vi "Andor_load_xml.vi"(8 "error in":errorcluster, 10 "child node in":refnum<k20>) -> (0 "error out":errorcluster, 2 "child node out":refnum<k20>, 3 "Andor settings":T1)   [LabVIEW 2012]
doc: "Loads HSDIO settings from xml. Expected format:\n\n<EnableHSDIOPulses>%b</EnableHSDIOPulses>\n<ResourceName>%s</ResourceName>\n<ClockRate>%f</ClockRate>\n<unitsPerSecond>%f</unitsPerSecond>\n<HardwareAlignmentQuantum units=\"samples\">%u</HardwareAlignmentQuantum>\n<ArrayOfScriptTriggers columns=\"id, source, type, edge, level\">\n<trigger>%s\\t%s\\t%s\\t%s\\t%s</trigger>\n</ArrayOfScriptTriggers>\n<ChannelsControl columns=\"Description, Active?, Idle State\">\n<channel>%s</channel>\n</ChannelsControl>\n<PulseGenerationScript>%s</PulseGenerationScript>\n<DirectoryToLookForWaveformFiles>%s</DirectoryToLookForWaveformFiles>\n<StartTrigger.WaitForStartTrigger>%b</StartTrigger.WaitForStartTrigger>\n<StartTrigger.source>%s</StartTrigger.source>\n<StartTrigger.edge>%s</StartTrigger.edge>\n\nMTL 2013 Jan 1"
uses:
  Camera/Andor/Andor_settings.ctl
  <vilib>/xml/Close Reference(Node).vi
  <resource>/objmgr/DOMUserDefRef.rc
  <vilib>/xml/NI_XML.lvlib
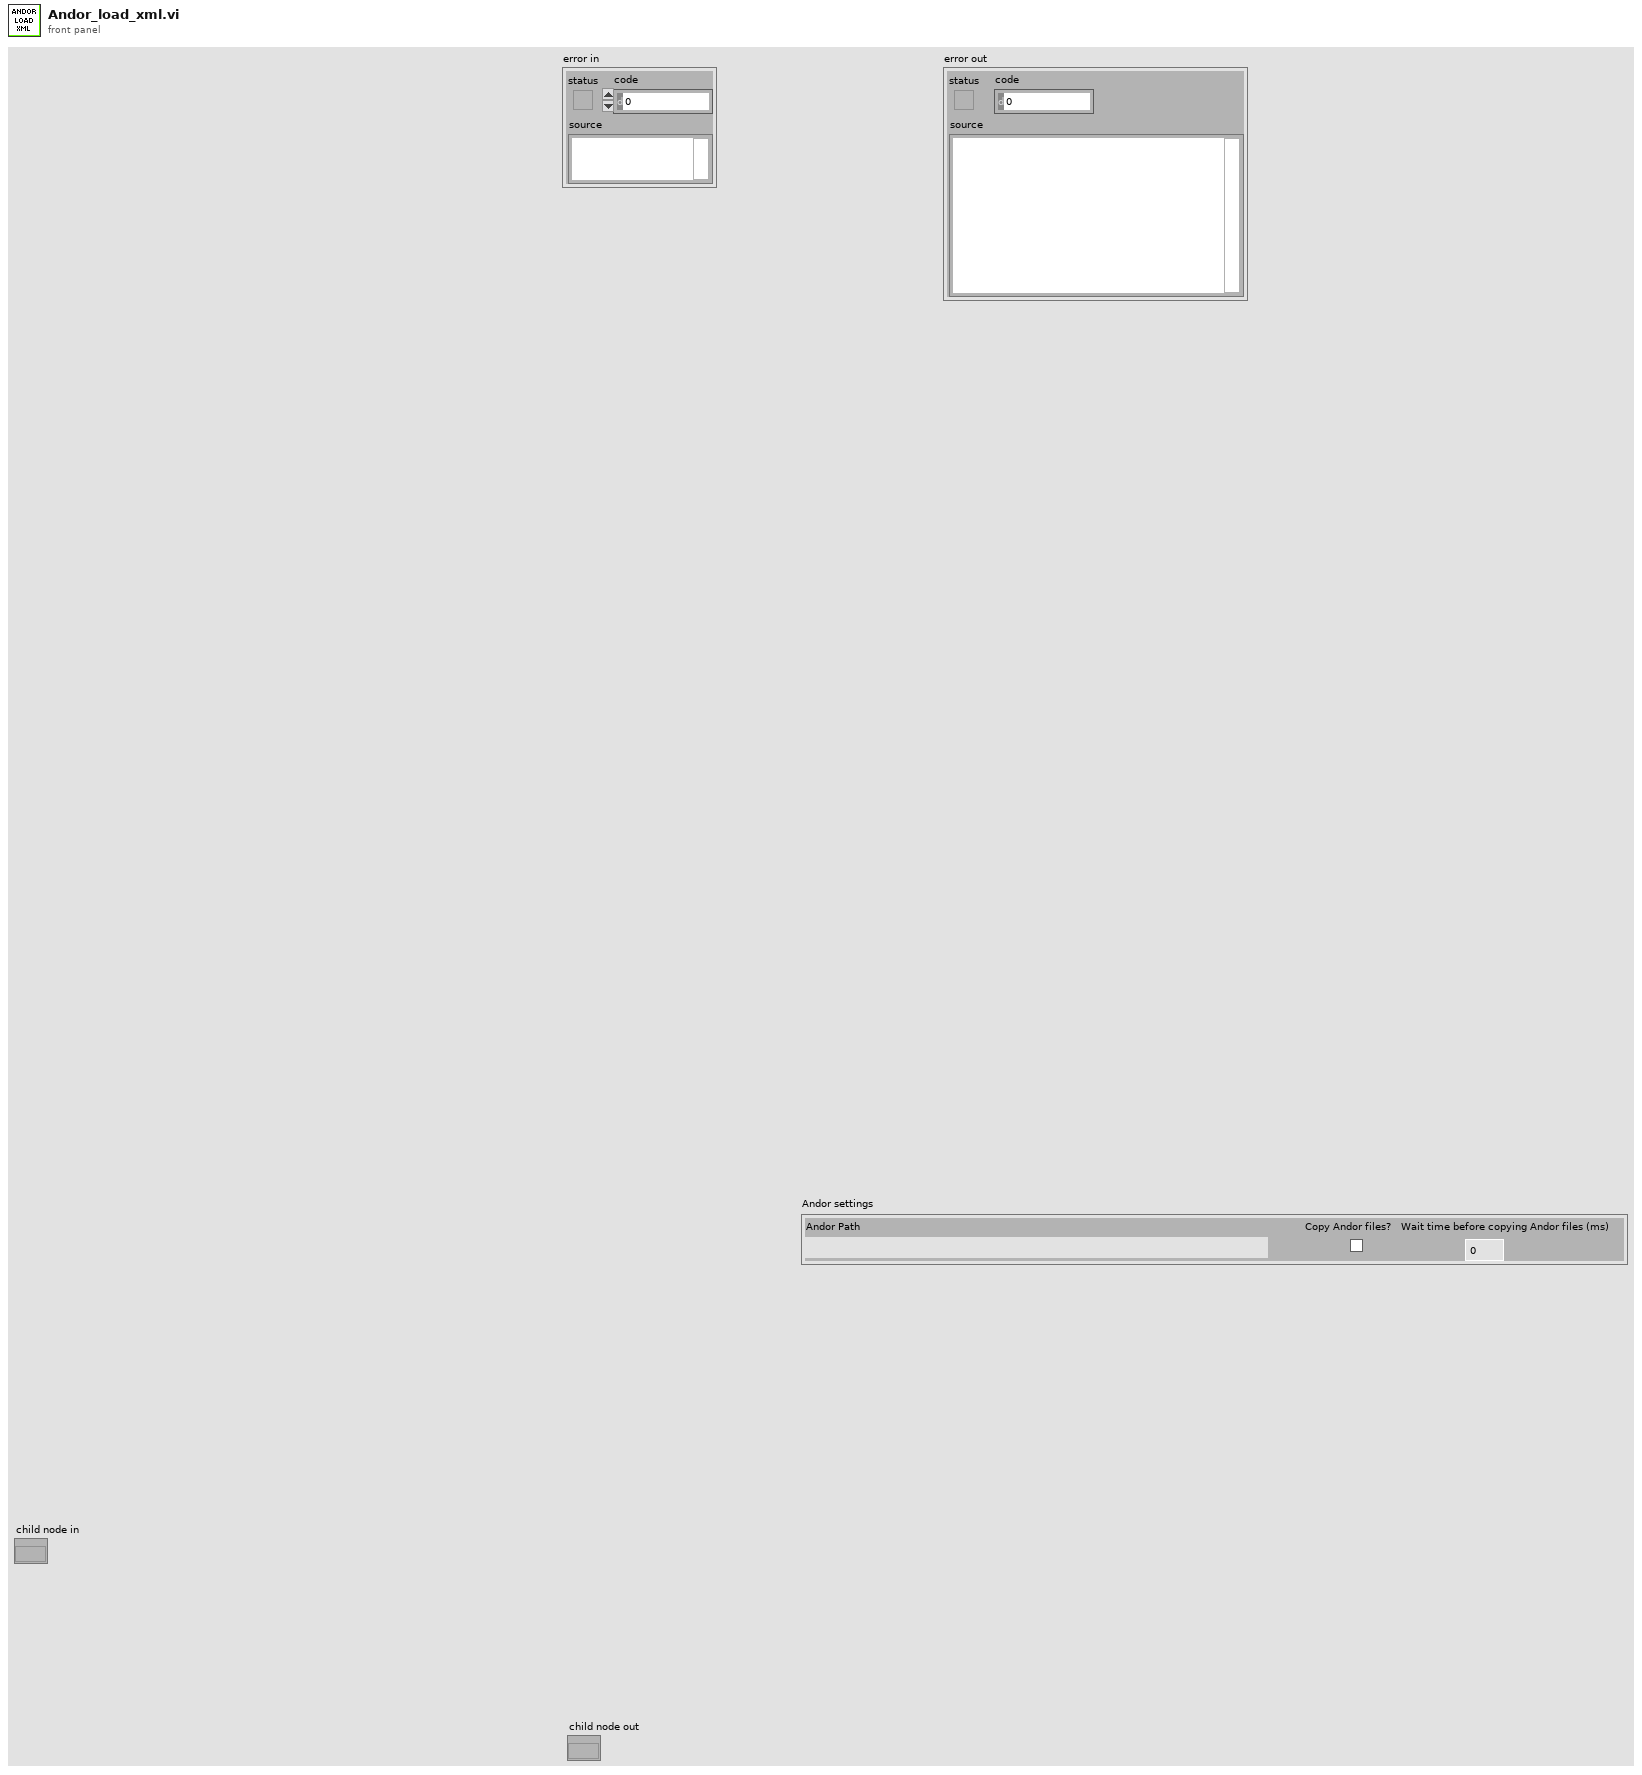
[diagram p1: front panel]
types:
  T1 = typedef "Andor_settings.ctl" = cluster{"Andor Path":path, "Copy any Andor files":bool, "Wait time before copying Andor files (ms)":u16}
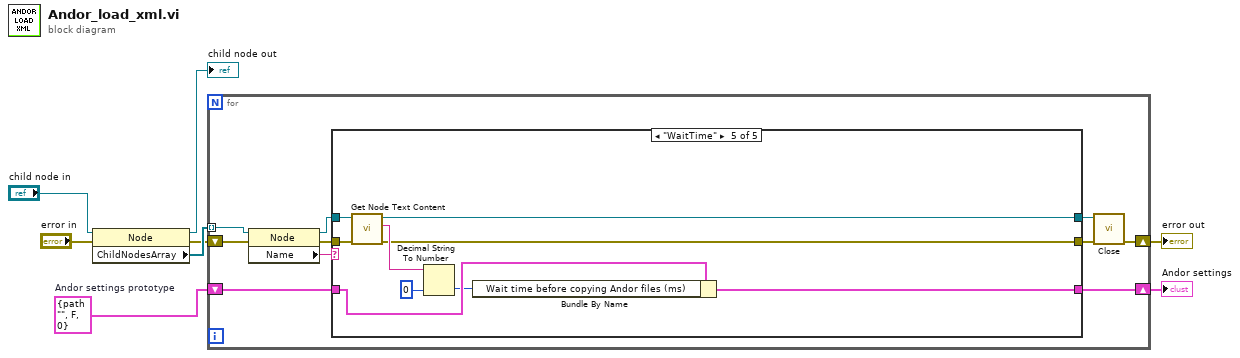
[diagram p0: block diagram]
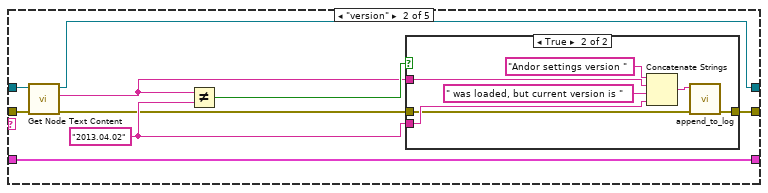
[diagram p3: hidden frame]
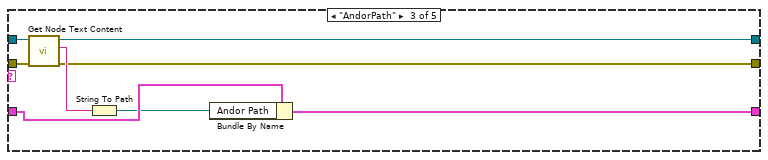
[diagram p5: hidden frame]
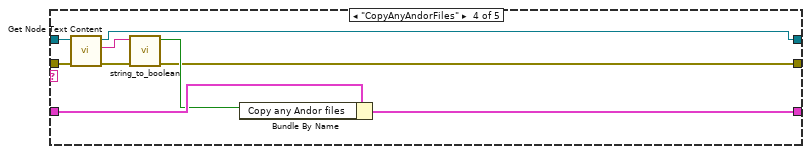
[diagram p6: hidden frame]
diagram:
  w2 = T1 {"Andor Path"=path "", "Copy any Andor files"=FALSE, "Wait time before copying Andor files (ms)"=0}  # Andor settings prototype
  n1 = property class="Node"(reference="child node in", error in="error in") -> (reference out=→"child node out":refnum<k20>, error out=w6:errorcluster, "ChildNodesArray"=w8:refnum<k20>[])
  n2 = for {
    tunnel: w8 -> [w10] mode=indexing
    shift-right: [w15] -> w1
    shift-left: w2 -> [w16]
    shift-right: [w12] -> w4
    shift-left: w6 -> [w9]
    n3 = property class="Node"(reference=w10, error in=w9) -> (reference out=w17:refnum<k20>, error out=w13:errorcluster, "Name"=w18:string)
    n4 = case shown="\"WaitTime\"" w18 {
      tunnel: w17 -> [w20 w26 w41 w54 w60]
      tunnel: w16 -> [w21 w24 w46 w52 w64]
      tunnel: [w21 w24 w45 w51 w63] -> w15
      tunnel: [w20 w23 w42 w55 w59] -> w14
      tunnel: w13 -> [w19 w25 w40 w53 w58]
      tunnel: [w19 w22 w39 w47 w57] -> w11
      frame "None", Default {
      }
      frame "version" {
        w28 = "2013.04.02" ("y")
        n5 = call <vilib>:"Get Node Text Content.vi"("error in (no error)"=w25, "node in"=w26) -> ("error out"=w27:errorcluster, "node text"=w29:string, "node out"=w23:refnum<k20>)  [unwired: 7 in]
        n6 = Not Equal?(x=w29, y=w28) -> (x != y?=w30:bool)
        n7 = case shown="True" w30 {
          tunnel: w29 -> [_ w37]
          tunnel: w28 -> [_ w35]
          tunnel: w27 -> [w31 w33]
          tunnel: [w31 w32] -> w22
          frame False {
          }
          frame True {
            n8 = Concatenate Strings("Andor settings version " ("string"), w37, " was loaded, but current version is " ("string"), w35) -> (w34:string)
            n9 = call "append_to_log.vi"("error in"=w33, "string"=w34) -> ("error out"=w32:errorcluster)  [unwired: 8 in, 1 out]
          }
        }
      }
      frame "AndorPath" {
        n10 = call <vilib>:"Get Node Text Content.vi"("error in (no error)"=w40, "node in"=w41) -> ("error out"=w39:errorcluster, "node text"=w44:string, "node out"=w42:refnum<k20>)  [unwired: 7 in]
        n11 = String To Path(string=w44) -> (path=w43:path)
        n12 = Bundle By Name(cluster=w46, "Andor Path"=w43) -> (w45:T1)
      }
      frame "CopyAnyAndorFiles" {
        n13 = call <vilib>:"Get Node Text Content.vi"("error in (no error)"=w53, "node in"=w54) -> ("error out"=w48:errorcluster, "node text"=w50:string, "node out"=w55:refnum<k20>)  [unwired: 7 in]
        n14 = call "string_to_boolean.vi"("error in"=w48, "string"=w50) -> ("error out"=w47:errorcluster, "boolean"=w49:bool)  [unwired: 8 in]
        n15 = Bundle By Name(cluster=w52, "Copy any Andor files"=w49) -> (w51:T1)
      }
      frame "WaitTime" {
        n16 = call <vilib>:"Get Node Text Content.vi"("error in (no error)"=w58, "node in"=w60) -> ("error out"=w57:errorcluster, "node text"=w62:string, "node out"=w59:refnum<k20>)  [unwired: 7 in]
        n17 = Decimal String To Number(string=w62, default (0L)=u16 0 ("default (0 I32)")) -> (number=w61:u16)  [unwired: 1 in, 1 out]
        n18 = Bundle By Name(cluster=w64, "Wait time before copying Andor files (ms)"=w61) -> (w63:T1)
      }
    }
    n19 = call-poly <vilib>:"Close.vi"("error in (no error)"=w11, "node"=w14) -> ("error out"=w12:errorcluster)  [unwired: 7 in]
  }
  "error out" <- w4
  "Andor settings" <- w1
